vi "SortidaAnalogicaUSB.vi"(0 "VelocitatAssaig":refnum<vi>, 1 "MotorActiu":refnum<vi>, 2 "MotorBipolar":refnum<vi>, 5 "stop":refnum<vi>, 7 "Pujar":refnum<vi>, 9 "Baixar":refnum<vi>, 11 "VelocitatRetorn":refnum<vi>, 12 "VelocitatMaxima":refnum<vi>, 13 "AssaigActiu":refnum<vi>) -> ()   [LabVIEW 2017]
uses:
  <vilib>/DAQmx/write.llb/DAQmx Write (Analog DBL 1Chan 1Samp).vi
  <vilib>/DAQmx/miscellaneous.llb/DAQmx Fill In Error Info.vi
  <resource>/objmgr/daqmx.rc
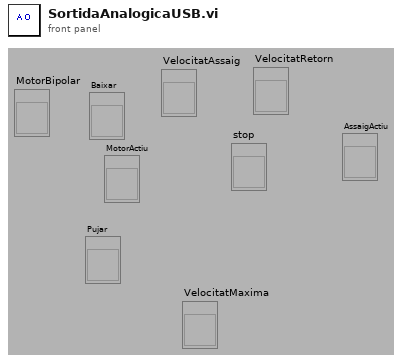
[diagram p1: front panel]
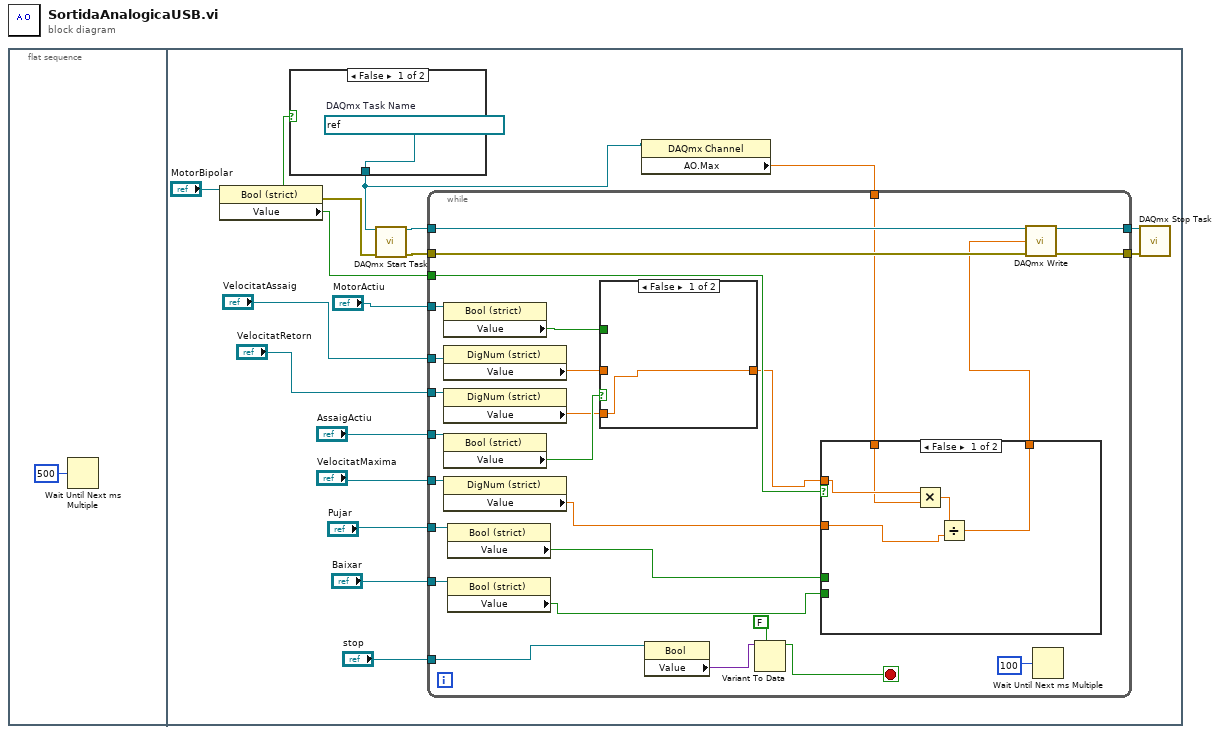
[diagram p0: block diagram]
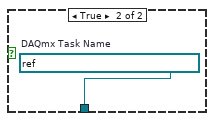
[diagram p2: hidden frame]
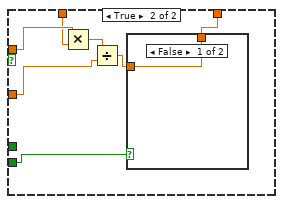
[diagram p3: hidden frame]
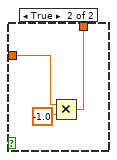
[diagram p4: hidden frame]
diagram:
  n1 = flat-sequence {
    frame #0 {
      n2 = Wait Until Next ms Multiple(millisecond multiple=u32 500) -> ()  [unwired: 1 out]
    }
    frame #1 {
      n3 = property class="Bool (strict)"(reference="MotorBipolar") -> (error out=w8:errorcluster, "Value"=w6:bool)  [unwired: 1 in, 1 out]
      n4 = case shown="False" w6 {
        tunnel: [w19 w20] -> w3
        frame False {
          w19 = refnum<k21> "Esclatometre_USBAnalogOut"  # DAQmx Task Name
        }
        frame True {
          w20 = refnum<k21> "Esclatometre_USBAnalogOut"  # DAQmx Task Name
        }
      }
      n5 = call <vilib>:"DAQmx Start Task.vi"("task/channels in"=w3, "error in"=w8) -> ("task out"=w18:refnum<k21>, "error out"=w16:errorcluster)  [unwired: 12 in]
      n6 = property class="DAQmx Channel"(reference=w3) -> ("AO.Max"=w2:dbl)  [unwired: 1 in, 2 out]
      n7 = while {
        tunnel: w18 -> [w32]
        tunnel: [w31] -> w17
        tunnel: w16 -> [w41]
        tunnel: [w47] -> w15
        tunnel: "stop" -> [w45]
        tunnel: "VelocitatAssaig" -> [w40]
        tunnel: "AssaigActiu" -> [w39]
        tunnel: "VelocitatMaxima" -> [w35]
        tunnel: "MotorActiu" -> [w34]
        tunnel: "Pujar" -> [w30]
        tunnel: "Baixar" -> [w29]
        tunnel: w6 -> [w28]
        tunnel: "VelocitatRetorn" -> [w22]
        tunnel: w2 -> [w21]
        stop <- w42 stop-if-true
        n8 = property class="Bool (strict)"(reference=w34) -> ("Value"=w33:bool)  [unwired: 1 in, 2 out]
        n9 = property class="DigNum (strict)"(reference=w40) -> ("Value"=w37:sgl)  [unwired: 1 in, 2 out]
        n10 = property class="DigNum (strict)"(reference=w22) -> ("Value"=w36:sgl)  [unwired: 1 in, 2 out]
        n11 = property class="Bool (strict)"(reference=w39) -> ("Value"=w38:bool)  [unwired: 1 in, 2 out]
        n12 = property class="DigNum (strict)"(reference=w35) -> ("Value"=w26:dbl)  [unwired: 1 in, 2 out]
        n13 = property class="Bool (strict)"(reference=w30) -> ("Value"=w24:bool)  [unwired: 1 in, 2 out]
        n14 = property class="Bool (strict)"(reference=w29) -> ("Value"=w23:bool)  [unwired: 1 in, 2 out]
        n15 = case shown="False" w38 {
          tunnel: [w64 w65] -> w27
          tunnel: w37 -> [_ w65]
          tunnel: w36 -> [w64 _]
          tunnel: w33 -> [_ _]
          frame False {
          }
          frame True {
          }
        }
        n16 = property class="Bool"(reference=w45) -> ("Value"=w44:variant)  [unwired: 1 in, 2 out]
        n17 = Variant To Data(type=FALSE ("stop"), Variant=w44) -> (data=w42:bool)  [unwired: 1 in, 1 out]
        n18 = case shown="False" w28 {
          tunnel: w27 -> [w51 w56]
          tunnel: w26 -> [w50 w55]
          tunnel: [w49 w57] -> w25
          tunnel: w24 -> [_ _]
          tunnel: w23 -> [_ w54]
          tunnel: w21 -> [w48 w53]
          frame False {
            n19 = Multiply(x=w51, y=w48) -> (x*y=w52:dbl)
            n20 = Divide(x=w52, y=w50) -> (x/y=w49:dbl)
          }
          frame True {
            n21 = Multiply(x=w56, y=w53) -> (x*y=w59:dbl)
            n22 = Divide(x=w59, y=w55) -> (x/y=w58:dbl)
            n23 = case shown="False" w54 {
              tunnel: w58 -> [w60 w62]
              tunnel: [w60 w61] -> w57
              frame False {
              }
              frame True {
                n24 = Multiply(x=w62, y=-1.0) -> (x*y=w61:dbl)
              }
            }
          }
        }
        n25 = call-poly <vilib>:"DAQmx Write.vi"("task/channels in"=w32, "data"=w25, "error in"=w41) -> ("task out"=w31:refnum<k21>, "error out"=w47:errorcluster)  [unwired: 10 in, 1 out]
        n26 = Wait Until Next ms Multiple(millisecond multiple=u32 100) -> ()  [unwired: 1 out]
      }
      n27 = call <vilib>:"DAQmx Stop Task.vi"("task/channels in"=w17, "error in"=w15) -> ()  [unwired: 12 in, 2 out]
    }
  }
